vi "Receive message by TOP.vi"(8 "error in (no error)":errorcluster, 9 "timeout (100)":i32=100, 11 "Mailbox in":T3) -> (0 "error out":errorcluster, 1 "timed out?":bool, 2 "Unread":i32, 3 "MSG packet":T1)   [LabVIEW 2018, in "MessengerLib.lvlib"]
uses:
  MessengerLib.lvlib
  Data types/MSG to TOP.ctl
  Data types/Module name.ctl
  Data types/Mailbox address.ctl
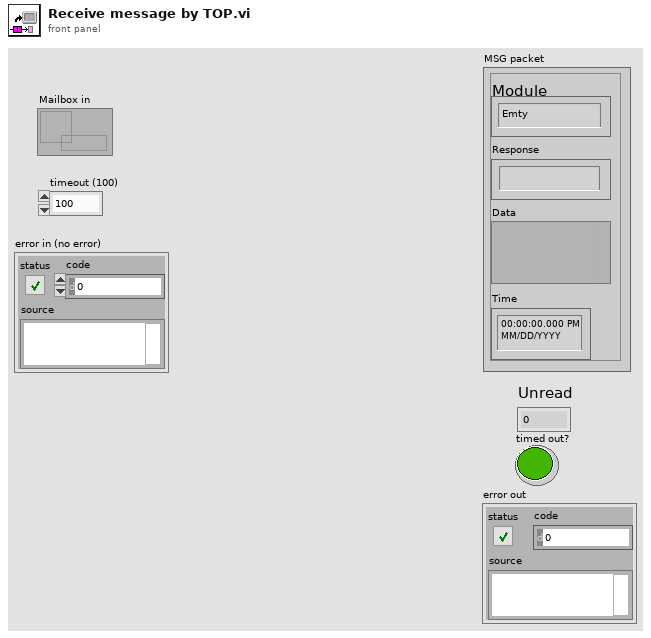
[diagram p1: front panel]
types:
  T1 = typedef "MessengerLib.lvlib/MSG to TOP.ctl" = cluster{"Module":T2, "Response":string, "Data":variant, "Time":timestamp}
  T2 = typedef "Module name.ctl" = enum16{"Emty", "Magnet", "VTI", "Excitation", "Servo", "Acquisition", "Rotator", "Digitizer", "SMU2450", "Carousel", "Multimeter", "Tmp monitor", "Power monitor"}
  T3 = typedef "MessengerLib.lvlib/Mailbox address.ctl" = refnum<queue>
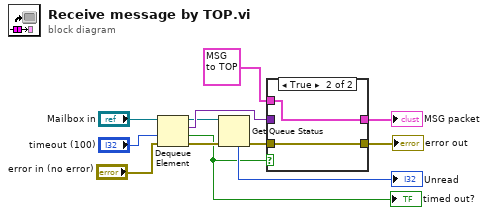
[diagram p0: block diagram]
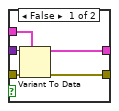
[diagram p2: hidden frame]
diagram:
  n1 = Dequeue Element(queue="Mailbox in", timeout in ms (-1)="timeout (100)", error in (no error)="error in (no error)") -> (queue out=w5:T3, element=w10:variant, timed out?=w1:bool, error out=w3:errorcluster)
  "timed out?" <- w1
  n2 = Get Queue Status(queue=w5, error in (no error)=w3) -> (error out=w4:errorcluster, # elements in queue=→"Unread":i32)  [unwired: 1 in, 6 out]
  n3 = case shown="True" w1 {
    tunnel: [w17 w19] -> w11
    tunnel: w10 -> [w16 _]
    tunnel: T1 {"Module"=enum."Emty", "Response"="", "Data"=variant, "Time"=timestamp(0 s since 1904-01-01)} ("MSG to UI") -> [w15 w18]
    tunnel: [w14 w18] -> w6
    tunnel: w4 -> [w13 w19]
    frame False {
      n4 = Variant To Data(error in=w13, type=w15, Variant=w16) -> (data=w14:T1, error out=w17:errorcluster)
    }
    frame True {
    }
  }
  "error out" <- w11
  "MSG packet" <- w6
